vi "PH_Timing.PC PU Delay.vi"(0 "i ref in":refnum<vi>, 1 "PU":T1, 2 "PU Delay":dbl, 5 "error in":errorcluster) -> (14 "i ref out":refnum<vi>, 19 "error out":errorcluster)   [LabVIEW 2014, in "PH_Timing.lvlib"]
doc: "This VI writes the incoming information to own attributes."
uses:
  PH_Timing.lvlib
  PH_Basics/PH_PP_Common/PH_PP_Common.PUs.ctl
  PH_Basics/PH_PP_Common/PH_PP_Common.lvlib
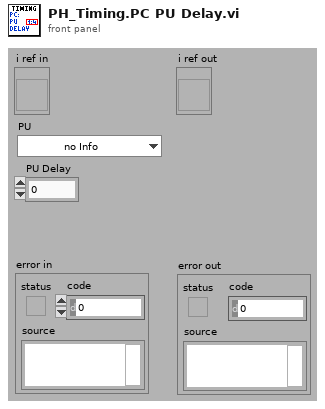
[diagram p1: front panel]
types:
  T1 = typedef "PH_PP_Common.lvlib/PH_PP_Common.PUs.ctl" = enum16{"no Info", "PA-19mm-1", "PA-19mm-2", "PA-45mm-PILC", "PA-45mm-MAIN", "MA-PU-1", "MA-PU-2", "MA-PU-3", "MA-PU-4", "MA-PU-5", "MA-PU-6", "MA-FR", "MA-PILC", "PA-45mm-DP"}
  T2 = typedef "PH_Timing.lvlib/PH_Timing.i attribute.ctl" = cluster{"Sequencer":cluster{"linked?":bool, "Proc State":string, "Ref State":refnum<vi>}, "Gate Generator":cluster{"GD":cluster{"Device Status":T3, "linked?":bool}, "Settings":T4, "GUI Ref":refnum<vi>}, "Interlock Bypass":cluster{"Instancename":string, "Switch linked?":bool, "Device Status":T3, "Ref Status":refnum<vi>}, "Roughtuner":cluster{"Settings":T5, "GUI Ref":refnum<vi>, "GD":cluster{"Device Status":T3, "linked?":bool}}, "0,5Hz Gater":cluster{"Settings":T6, "GUI Ref":refnum<vi>, "GD":cluster{"Device Status":T3, "linked?":bool}}, "Slow Trigger":cluster{"Settings":T7, "GUI Ref":refnum<vi>, "Service ID Delay":i32, "Service ID Ext Trig":i32, "Wanted Settings":T7}, "Timing Mode":cluster{"Mode":T8, "GUI Ref":refnum<vi>, "Service ID T2":i32, "Service ID Mode":i32, "Wanted Mode":T8}, "ns Generator":cluster{"Settings":T9, "ns Generator Settings":refnum<vi>, "GD":cluster{"Device Status":T3, "linked?":bool}}, "Phase FEs":cluster{"Settings":T12, "GUI Ref":refnum<vi>, "Service ID Phase":i32, "Wanted Settings":T12}, "GD GUI Refs":refnum<vi>[], "Heads":T13[], "GUI Ref Delete":refnum<vi>}
  T3 = typedef "PH_StatusHandler.lvlib/PH_StatusHandler.Status.ctl" = i16
  T4 = typedef "PH_Timing.lvlib/PH_Timing.GateGen.ctl" = cluster{"Instance":string, "Channel Gate":i32, "Channel T2":i32, "Width Gate":dbl, "Width T2":dbl, "Delay Gate":dbl, "Delay T2":dbl, "Gate activ":bool, "T2 activ":bool, "System Mode":enum16{"Normal", "Single", "Burst", "Duty Cycle"}}
  T5 = typedef "PH_Timing.lvlib/PH_Timing.Roughtuner.ctl" = cluster{"Instance":string, "Phase PHELIX / UNILAC":cluster{"Channel":u16, "relative to":u16, "Delay [ms]":dbl}, "Pulse Length":cluster{"Channel":u16, "relative to":u16, "Delay [ms]":dbl}, "Trigger":cluster{"externally?":bool, "Rate [Hz]":dbl}}
  T6 = typedef "PH_Timing.lvlib/PH_Timing.0.5HzGater.ctl" = cluster{"Instance":string, "Channel ns FE Delay":i32, "Channel 0.5Hz":i32, "Width ns FE Delay":dbl, "Width 0.5Hz":dbl, "Delay ns FE Delay":dbl, "Delay 0.5Hz":dbl, "ns FE Delay active":bool, "0.5Hz activ":bool, "ns FE Delay inverted":bool, "0.5Hz inverted":bool}
  T7 = typedef "PH_Timing.lvlib/PH_Timing.Slow Trigger Settings.ctl" = cluster{"Delay":dbl, "externally triggered?":bool}
  T8 = typedef "PH_Timing.lvlib/PH_Timing.Timing Mode.ctl" = cluster{"T2":i16, "Modeselector":enum32{"10 Hz", "0.5 Hz", "Shot"}}
  T9 = typedef "PH_Timing.lvlib/PH_Timing.ns Generator.ctl" = cluster{"Instance":string, "Phase fs / ns FE":cluster{"Channel":T10, "Settings":T11}}
  T10 = typedef "Stanford Research DG645 - Driver.lvlib/Channel.ctl" = i32
  T11 = typedef "PH_SRDG645.lvlib/PH_SRDG645.Channel Settings.ctl" = cluster{"Delay [s]":dbl, "relative to":i32}
  T12 = typedef "PH_Timing.lvlib/PH_Timing.Phase FEs.ctl" = cluster{"Phase":dbl}
  T13 = typedef "PH_Timing.lvlib/PH_Timing.PU Data.ctl" = cluster{"linked?":bool, "Data":T14, "GD":cluster{"Device Status":T3, "linked?":bool}, "GUI Ref":refnum<vi>, "PU":T1}
  T14 = typedef "PH_Timing.lvlib/PH_Timing.PU Info.ctl" = cluster{"Act CH?":bool, "GD":string, "CH":i32, "Delay":dbl, "active":bool, "in Use?":bool}
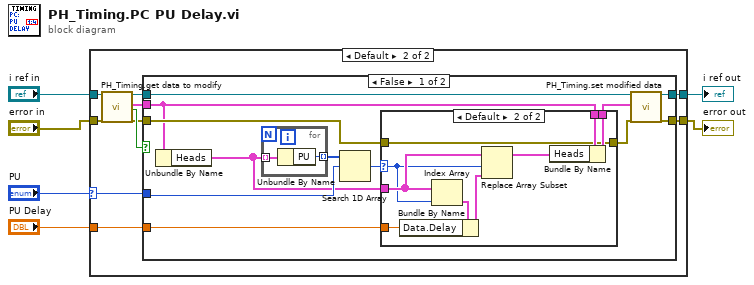
[diagram p0: block diagram]
diagram:
  n1 = case shown="Default" "PU" {
    selector: "PU" -> [_ w9]
    tunnel: [w7 w16] -> w6
    tunnel: "error in" -> [w7 w14]
    tunnel: [w8 w13] -> w4
    tunnel: "i ref in" -> [w8 w11]
    tunnel: "PU Delay" -> [_ w10]
    frame "no Info" {
    }
    frame Default {
      n2 = call "PH_Timing.get data to modify.vi"("i ref in"=w11, "error in (no error)"=w14) -> ("i ref out"=w12:refnum<vi>, "i attribute"=w17:T2, "timed out"=w18:bool, "error out"=w15:errorcluster)  [unwired: 14 in]
      n3 = case shown="False" w18 {
        tunnel: w12 -> [w30 w45]
        tunnel: [w29 w45] -> w13
        tunnel: w15 -> [w26 w44]
        tunnel: [w28 w44] -> w16
        tunnel: w17 -> [w24 _]
        tunnel: w9 -> [w20 _]
        tunnel: w10 -> [w21 _]
        frame False {
          n4 = Unbundle By Name(w24) -> ("Heads"=w19:T13[])
          n5 = for {
            tunnel: w19 -> [w43] mode=indexing
            tunnel: [w42] -> w27 mode=indexing
            n6 = Unbundle By Name(w43) -> ("PU"=w42:T1)
          }
          n7 = Search 1D Array(1D array=w27, element=w20) -> (index of element=w22:i32)  [unwired: 1 in]
          n8 = case shown="Default" w22 {
            selector: w22 -> [_ w36]
            tunnel: w26 -> [w32 w34]
            tunnel: [w32 w34] -> w25
            tunnel: w21 -> [_ w35]
            tunnel: w24 -> [w31 w41]
            tunnel: [w31 w40] -> w23
            tunnel: w19 -> [_ w38]
            frame -1 {
            }
            frame Default {
              n9 = Index Array(array=w38, index=w36) -> (element=w39:T13)
              n10 = Bundle By Name(cluster=w39, "Data.Delay"=w35) -> (w37:T13)
              n11 = Replace Array Subset(array=w38, new element=w37, index=w36) -> (w33:T13[])
              n12 = Bundle By Name(cluster=w41, "Heads"=w33) -> (w40:T2)
            }
          }
          n13 = call "PH_Timing.set modified data.vi"("i ref in"=w30, "i attribute"=w23, "error in (no error)"=w25) -> ("i ref out"=w29:refnum<vi>, "error out"=w28:errorcluster)  [unwired: 15 in]
        }
        frame True {
        }
      }
    }
  }
  "error out" <- w6
  "i ref out" <- w4
